vi "Sort_Alpha_Order.vi"(0 "Split_Data":string[](array[string]), 11 "Error_In":errorcluster, 12 "Order (Z to A)":T1) -> (4 "Sorted_Array":string[](array[string]), 15 "Error_Out":errorcluster)   [LabVIEW 2021, in "Custom_Sort_Library.lvlib"]
doc: "This VI Sort the data in the required reverse alpha-order"
uses:
  Custom_Sort_Library.lvlib
  Library_Controls/Order (Z to A).ctl
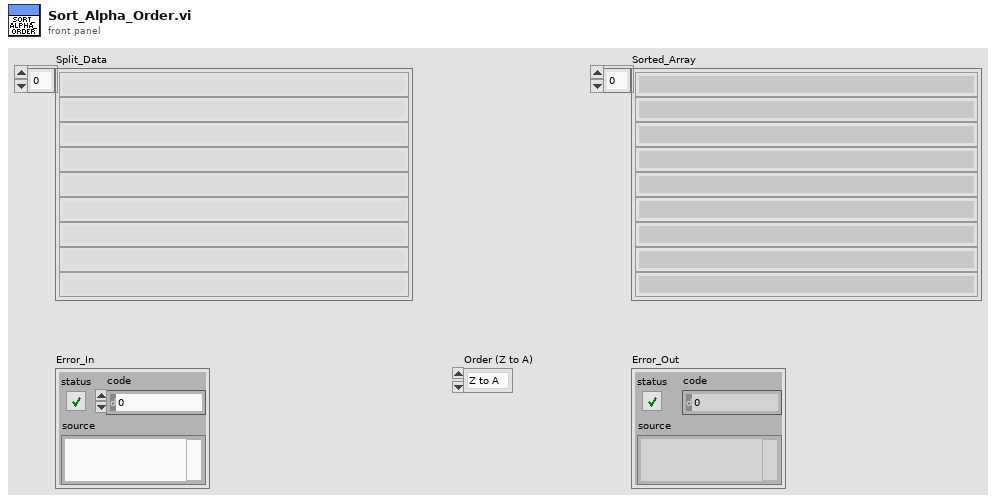
[diagram p1: front panel]
types:
  T1 = typedef "Custom_Sort_Library.lvlib/Order (Z to A).ctl" = enum16{"Z to A", "A to Z"}
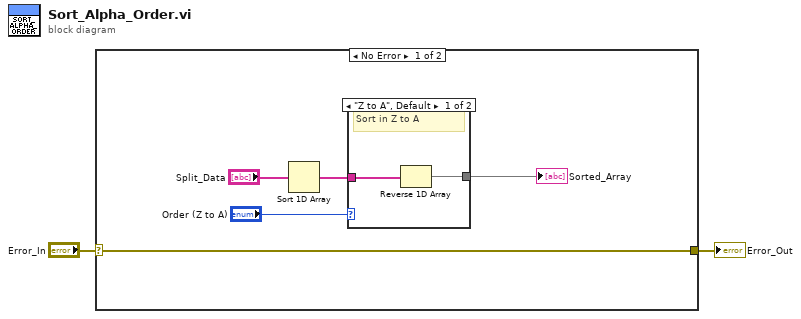
[diagram p0: block diagram]
diagram:
  n1 = case shown="No Error" "Error_In" {
    selector: "Error_In" -> [w4 w11]
    tunnel: [w4 w11] -> w1
    frame No Error {
      n2 = Sort 1D Array(array="Split_Data") -> (sorted array=w7:string[])
      n3 = case shown="\"Z to A\", Default" "Order (Z to A)" {
        tunnel: w7 -> [w9 w10]
        tunnel: [w8 w10] -> w6
        frame "Z to A", Default {
          # "Sort in Z to A"
          n4 = Reverse 1D Array(array=w9) -> (reversed array=w8:string[])
        }
        frame "A to Z" {
          # "Sort in A to Z"
        }
      }
      "Sorted_Array" <- w6
    }
    frame Error {
    }
  }
  "Error_Out" <- w1
